vi "Update UI.vi"(8 "error in (no error)":errorcluster, 10 "DataExchange":T1, 11 "Controller Template in":refnum<class "Displayer.lvclass">) -> (0 "error out":errorcluster, 3 "Controller Template out":refnum<class "Displayer.lvclass">)   [LabVIEW 2020, in "Displayer.lvlib" / "Displayer.lvclass"]
uses:
  Displayer.lvclass
  Model/Hardware Abstraction Layer/Component/Device/Device/DataExchange.ctl
  Displayer.lvclass/Displayer.ctl
  Interface/DataListener/DataListener.lvclass
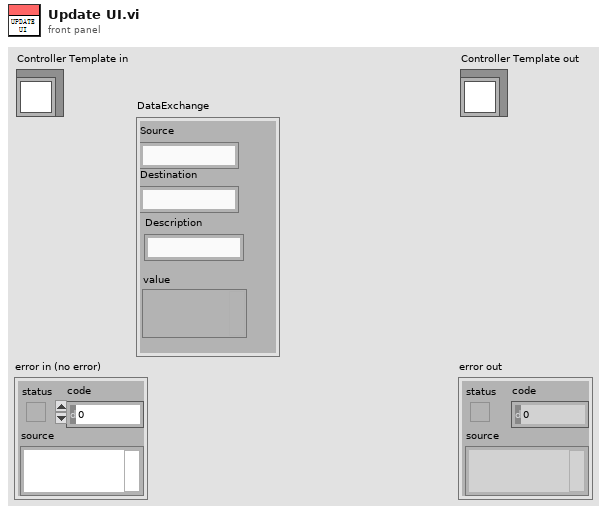
[diagram p1: front panel]
types:
  T1 = typedef "DataListener.lvclass/DataExchange.ctl" = cluster{"Source":string, "Destination":string, "Description":string, "value":variant}
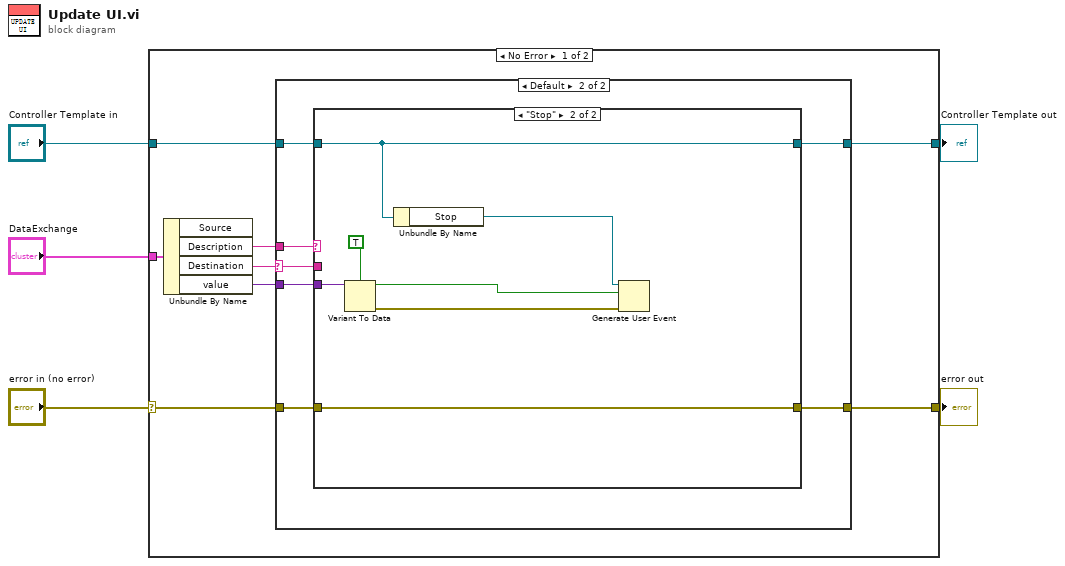
[diagram p0: block diagram]
diagram:
  n1 = case shown="No Error" "error in (no error)" {
    selector: "error in (no error)" -> [w8 w33]
    tunnel: [w7 w33] -> w4
    tunnel: [w9 w32] -> w2
    tunnel: "Controller Template in" -> [w10 w32]
    tunnel: "DataExchange" -> [w13 _]
    frame No Error {
      n2 = Unbundle By Name(w13) -> ("Description"=w11:string, "Destination"=w6:string, "value"=w12:variant)  [unwired: 1 out]
      n3 = case shown="Default" w6 {
        selector: w6 -> [_ w16]
        tunnel: w12 -> [_ w22]
        tunnel: w11 -> [_ w21]
        tunnel: w10 -> [w15 w20]
        tunnel: [w15 w19] -> w9
        tunnel: w8 -> [w14 w18]
        tunnel: [w14 w17] -> w7
        frame "duplicate this case" {
        }
        frame Default {
          n4 = case shown="\"Stop\"" w21 {
            tunnel: w22 -> [_ w31]
            tunnel: [w24 w26] -> w19
            tunnel: w20 -> [w24 w26]
            tunnel: [w23 w25] -> w17
            tunnel: w18 -> [w23 w25]
            tunnel: w16 -> [_ _]
            frame Default {
            }
            frame "Stop" {
              n5 = Variant To Data(type=TRUE, Variant=w31) -> (data=w29:bool, error out=w27:errorcluster)  [unwired: 1 in]
              n6 = Unbundle By Name(w26) -> ("Stop"=w30:refnum<user-event>)
              n7 = Generate User Event(user event=w30, event data cluster=w29, error in=w27) -> ()  [unwired: 1 in, 2 out]
            }
          }
        }
      }
    }
    frame Error {
    }
  }
  "error out" <- w4
  "Controller Template out" <- w2
